vi "SQL_DeleteData.vi"(5 "To Delete":string, 7 "Column Name":string, 8 "error in (no error)":errorcluster, 10 "Table":string, 11 "SQL in":refnum<class "SQL.lvclass">) -> (0 "error out":errorcluster, 3 "SQL out":refnum<class "SQL.lvclass">)   [LabVIEW 2012, in "SQL.lvclass"]
uses:
  SQL.lvclass
  <vilib>/addons/database/NI_Database_API.lvlib
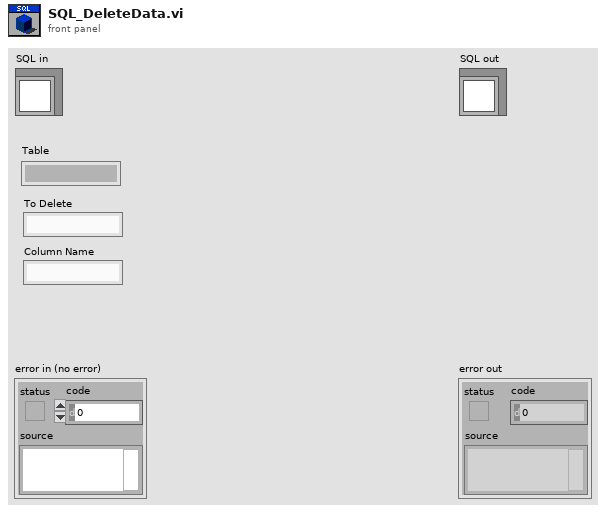
[diagram p1: front panel]
types:
  T1 = typedef "SQL.lvclass/ObjectAttributes.ctl" = cluster{"DB Connection Reference":T2}
  T2 = typedef "NI_Database_API.lvlib/Conn ObjectReference.ctl" = refnum<k1>
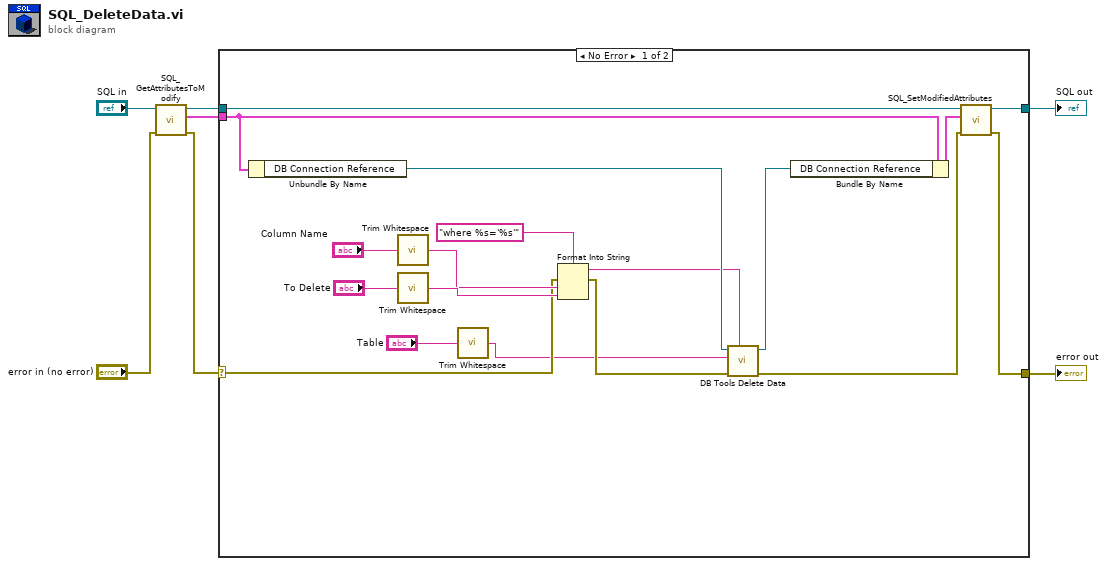
[diagram p0: block diagram]
diagram:
  n1 = call "SQL_GetAttributesToModify.vi"("error in (no error)"="error in (no error)", "reference in"="SQL in") -> ("error out"=w1:errorcluster, "Attributes"=w3:T1, "reference out"=w4:refnum<class "SQL.lvclass">)  [unwired: 6 in, 1 out]
  n2 = case shown="No Error" w1 {
    selector: w1 -> [w12 w27]
    tunnel: [w22 w27] -> w7
    tunnel: [w24 w26] -> w6
    tunnel: w4 -> [w25 w26]
    tunnel: w3 -> [w21 _]
    frame No Error {
      n3 = Unbundle By Name(w21) -> ("DB Connection Reference"=w13:T2)
      n4 = call <vilib>:"Trim Whitespace.vi"("string"="Column Name") -> ("trimmed string"=w17:string)  [unwired: 1 in]
      n5 = call <vilib>:"Trim Whitespace.vi"("string"="To Delete") -> ("trimmed string"=w18:string)  [unwired: 1 in]
      n6 = call <vilib>:"Trim Whitespace.vi"("string"="Table") -> ("trimmed string"=w10:string)  [unwired: 1 in]
      n7 = Format Into String(format string="where %s='%s'", error in=w12, w17, w18) -> (resulting string=w8:string, error out=w11:errorcluster)  [unwired: 1 in]
      n8 = call <vilib>:"DB Tools Delete Data.vi"("condition"=w8, "error in (no error)"=w11, "table"=w10, "connection reference"=w13) -> ("error out"=w23:errorcluster, "connection reference out"=w19:T2)  [unwired: 6 in]
      n9 = Bundle By Name(cluster=w21, "DB Connection Reference"=w19) -> (w20:T1)
      n10 = call "SQL_SetModifiedAttributes.vi"("error in (no error)"=w23, "Attributes"=w20, "reference in"=w25) -> ("error out"=w22:errorcluster, "reference out"=w24:refnum<class "SQL.lvclass">)  [unwired: 7 in]
    }
    frame Error {
    }
  }
  "error out" <- w7
  "SQL out" <- w6
